vi "GetMinMaxFromFile.vi"(5 "error in (no error)":errorcluster) -> (16 "MinMaxData":T1, 19 "error out":errorcluster)   [LabVIEW 2014, in "IndoorData.lvclass"]
uses:
  IndoorData.lvclass
  MinMaxData.ctl
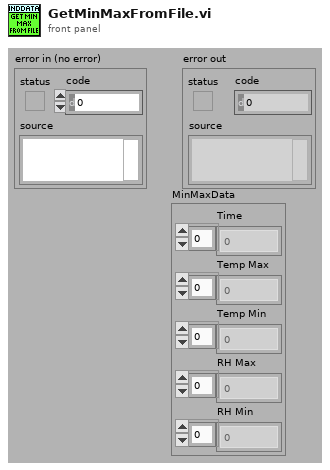
[diagram p1: front panel]
types:
  T1 = typedef "IndoorData.lvclass/MinMaxData.ctl" = cluster{"Time":dbl[], "Temp Max":dbl[], "Temp Min":dbl[], "RH Max":dbl[], "RH Min":dbl[]}
  T2 = typedef "IndoorData.lvclass/ObjectAttributes.ctl" = cluster{"DebugData":T3, "Actual":T4, "BufferedReadings":T5, "AVGReadings":T5, "LogFolder":path, "FirstLog?":bool, "MinMaxFile":path}
  T3 = typedef "IndoorData.lvclass/DebugData.ctl" = cluster{"Rev":string, "Location":string, "LoopIdx":i32, "PiCoreTemp":dbl, "Error":errorcluster}
  T4 = typedef "IndoorData.lvclass/ActualValues.ctl" = cluster{"Time":dbl, "Temp":dbl, "RH":dbl}
  T5 = typedef "IndoorData.lvclass/BufferedReadings.ctl" = cluster{"Time":dbl[], "Temp":dbl[], "RH":dbl[]}
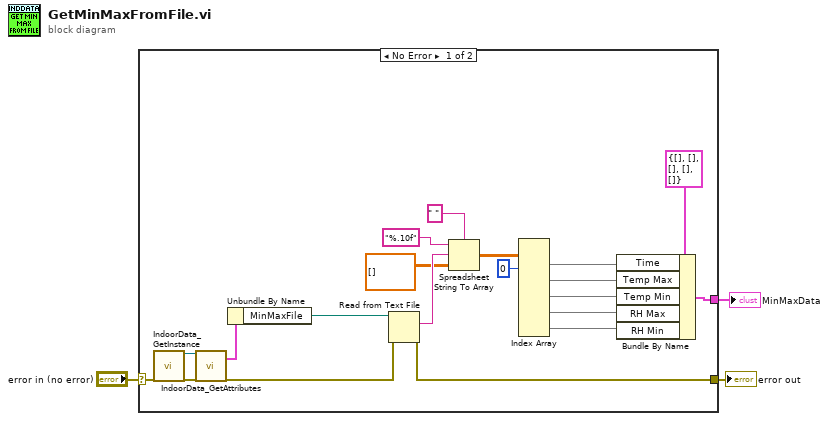
[diagram p0: block diagram]
diagram:
  n1 = case shown="No Error" "error in (no error)" {
    selector: "error in (no error)" -> [w12 w24]
    tunnel: [w9 w24] -> w2
    tunnel: [w8 _] -> w1
    frame No Error {
      n2 = call "IndoorData_GetInstance.vi"("error in (no error)"=w12) -> ("reference out"=w14:refnum<class "IndoorData.lvclass">, "error out"=w11:errorcluster)  [unwired: 14 in, 3 out]
      n3 = call "IndoorData_GetAttributes.vi"("reference in"=w14, "error in (no error)"=w11) -> ("Data"=w13:T2, "error out"=w10:errorcluster)  [unwired: 14 in, 2 out]
      n4 = Unbundle By Name(w13) -> ("MinMaxFile"=w7:path)
      n5 = Read from Text File(file (use dialog)=w7, error in=w10) -> (text=w23:string, error out=w9:errorcluster)  [unwired: 2 in, 2 out]
      n6 = Spreadsheet String To Array(delimiter (Tab)=" ", format string="%.10f", spreadsheet string=w23, array type (2D Dbl)=dbl[][] []) -> (array=w19:dbl[][])
      n7 = Index Array(array=w19, index (col) #1=0 ("disabled index (col)")) -> (element #1=w17:dbl[], element #2=w16:dbl[], element #3=w15:dbl[], element #4=w5:dbl[], element #5=w4:dbl[])  [unwired: 9 in]
      n8 = Bundle By Name(cluster=T1 {"Time"=[], "Temp Max"=[], "Temp Min"=[], "RH Max"=[], "RH Min"=[]} ("Cluster"), "Time"=w17, "Temp Max"=w16, "Temp Min"=w15, "RH Max"=w5, "RH Min"=w4) -> (w8:T1)
    }
    frame Error {
    }
  }
  "error out" <- w2
  "MinMaxData" <- w1
